vi "DisplayName.vi"(1 "State In":T1) -> (0 "Name":string)   [LabVIEW 2018, in "Shuffle Array.xnode"]
doc: "This ability is deprecated; prefer GetDisplayName2.\n\nThis ability VI is used to supply LabVIEW with the name of your XNode. This is used as the default value for the label, it is used to mark entries in the error list and the difference list.\n\nDefault behavior: None.\n\nThis ability does not provide UI and OS messages are not handled."
uses:
  Shuffle Array.xnode
  State.ctl
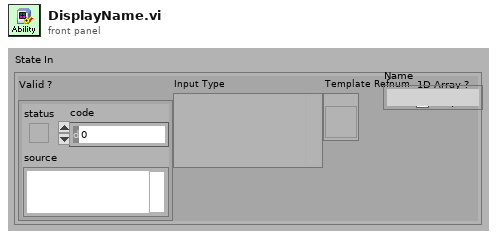
[diagram p1: front panel]
types:
  T1 = typedef "Shuffle Array.xnode/State.ctl" = cluster{"Valid ?":errorcluster, "Input Type":variant, "Template Refnum":refnum<vi>, "1D Array ?":bool}
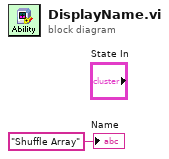
[diagram p0: block diagram]
diagram:
  "Name" <- "Shuffle Array" ("Name")
